vi "Get All Aliases.vi"(8 "error in (no error)":errorcluster, 11 "Aliases Ref in":T2 format="%.0x") -> (0 "error out":errorcluster, 1 "Aliases found":bool, 2 "All Alias Mappings":T1[](array[typedef]), 3 "Aliases Ref out":T2 format="%.0x")   [LabVIEW 2017, in "Switch Scripting.lvlib"]
uses:
  Switch Scripting.lvlib
  <vilib>/NI Veristand/Custom Device API/Custom Device Item Ref.ctl
  Routing Channel/Alias Mapping.ctl
  <vilib>/NI Veristand/Custom Device API/Get Item Property (String).vi
  <vilib>/NI VeriStand/Custom Device API/Custom Device API.lvlib
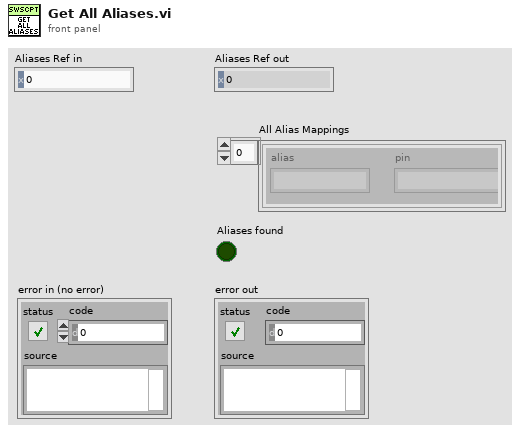
[diagram p1: front panel]
types:
  T1 = typedef "Switch Scripting.lvlib/Alias Mapping.ctl" = cluster{"alias":string, "pin":string}
  T2 = typedef "Custom Device API.lvlib/Custom Device Item Ref.ctl" = u64
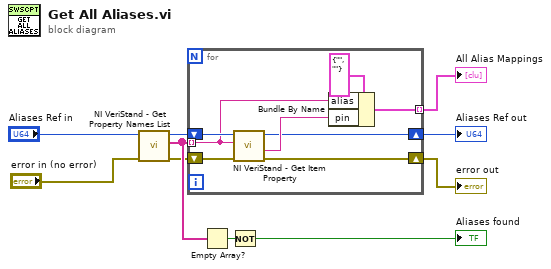
[diagram p0: block diagram]
diagram:
  n1 = call <vilib>:"NI VeriStand - Get Property Names List.vi"("error in (no error)"="error in (no error)", "Item Ref in"="Aliases Ref in") -> ("error out"=w7:errorcluster, "Property Names"=w8:string[], "Item Ref out"=w2:T2)  [unwired: 7 in]
  n2 = for {
    tunnel: w8 -> [w14] mode=indexing
    shift-right: [w16] -> w4
    shift-left: w7 -> [w18]
    tunnel: [w12] -> w5 mode=indexing
    shift-right: [w11] -> w1
    shift-left: w2 -> [w17]
    n3 = call-poly <vilib>:"NI VeriStand - Get Item Property.vi"("error in (no error)"=w18, "Property Name"=w14, "Item Ref in"=w17) -> ("error out"=w16:errorcluster, "Value"=w13:string, "Item Ref out"=w11:T2)  [unwired: 5 in, 1 out]
    n4 = Bundle By Name(cluster=T1 {"alias"="", "pin"=""} ("Connection"), "alias"=w14, "pin"=w13) -> (w12:T1)
  }
  "error out" <- w4
  "Aliases Ref out" <- w1
  "All Alias Mappings" <- w5
  n5 = Empty Array?(array=w8) -> (empty?=w10:bool)
  n6 = Not(x=w10) -> (.not. x?=→"Aliases found":bool)
